vi "normalize128_servo.vi"(4 "D":dbl, 5 "C":dbl, 6 "B":dbl, 7 "A":dbl) -> (0 "mD":dbl, 1 "mC":dbl, 2 "mB":dbl, 3 "mA":dbl)   [LabVIEW 2010, in "LASA Beta.lvrbt"]
doc: "Converts the FTC Controller (values from -127 to 127) to a HiTechnic readable servo LOCATION value from 0 to 255."
uses:
  LASA Beta.lvrbt
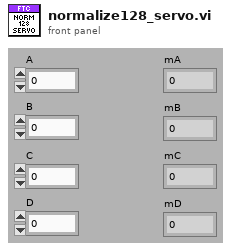
[diagram p1: front panel]
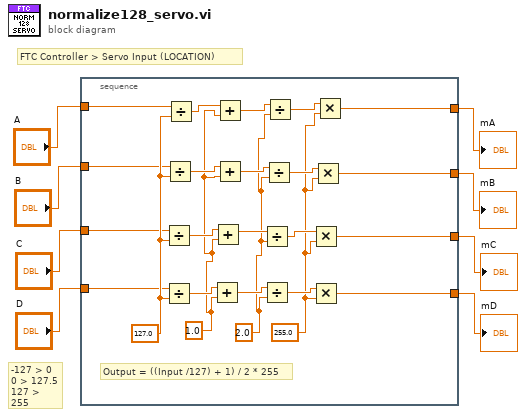
[diagram p0: block diagram]
diagram:
  # "-127 > 0\n0 > 127.5 \n127 > 255"
  # "FTC Controller > Servo Input (LOCATION)"
  n1 = stacked-sequence {
    tunnel: "A" -> [w31]
    tunnel: "B" -> [w30]
    tunnel: "C" -> [w29]
    tunnel: "D" -> [w28]
    tunnel: [w12] -> w4
    tunnel: [w11] -> w3
    tunnel: [w10] -> w2
    tunnel: [w9] -> w1
    frame #0 {
      w13 = 255.0 ("y")
      w18 = 2.0 ("y")
      w23 = 1.0 ("y")
      w32 = 127.0 ("y")
      # "Output = ((Input /127) + 1) / 2 * 255"
      n2 = Divide(x=w29, y=w32) -> (x/y=w25:dbl)
      n3 = Divide(x=w28, y=w32) -> (x/y=w24:dbl)
      n4 = Divide(x=w30, y=w32) -> (x/y=w26:dbl)
      n5 = Divide(x=w31, y=w32) -> (x/y=w27:dbl)
      n6 = Add(x=w24, y=w23) -> (x+y=w19:dbl)
      n7 = Add(x=w25, y=w23) -> (x+y=w20:dbl)
      n8 = Add(x=w27, y=w23) -> (x+y=w21:dbl)
      n9 = Add(x=w26, y=w23) -> (x+y=w22:dbl)
      n10 = Divide(x=w20, y=w18) -> (x/y=w16:dbl)
      n11 = Divide(x=w19, y=w18) -> (x/y=w17:dbl)
      n12 = Divide(x=w22, y=w18) -> (x/y=w15:dbl)
      n13 = Divide(x=w21, y=w18) -> (x/y=w14:dbl)
      n14 = Multiply(x=w16, y=w13) -> (x*y=w10:dbl)
      n15 = Multiply(x=w17, y=w13) -> (x*y=w9:dbl)
      n16 = Multiply(x=w15, y=w13) -> (x*y=w11:dbl)
      n17 = Multiply(x=w14, y=w13) -> (x*y=w12:dbl)
    }
  }
  "mA" <- w4
  "mB" <- w3
  "mC" <- w2
  "mD" <- w1
